vi "ELVIS III v1.0 Build MUX Configuration AI Continuous.vi"(11 "AI (Continuous) Channels List":T4) -> (2 "Bank Count":u8[](array[numeric]), 3 "Channel Reservation Info":T1)   [LabVIEW 2021]
uses:
  <vilib>/myRIO/Common/Instrument Driver Framework/ELVIS III v1.0/AI Continuous/typedefs/AI Continuous Channels List.ctl
  <vilib>/myRIO/Common/Instrument Driver Framework/ELVIS III v1.0/AI Continuous/typedefs/ELVIS III v1.0 AI Continuous Channels Enum.ctl
  <vilib>/myRIO/Common/Instrument Driver Framework/ELVIS III v1.0/Resource Manager/typedefs/ELVIS III v1.0 Channel Reservation List.ctl
  <vilib>/myRIO/Common/Instrument Driver Framework/ELVIS III v1.0/Resource Manager/typedefs/ELVIS III v1.0 Channel Reservation Info.ctl
  <vilib>/myRIO/Common/Instrument Driver Framework/ELVIS III v1.0/Resource Manager/typedefs/ELVIS III v1.0 Connector List.ctl
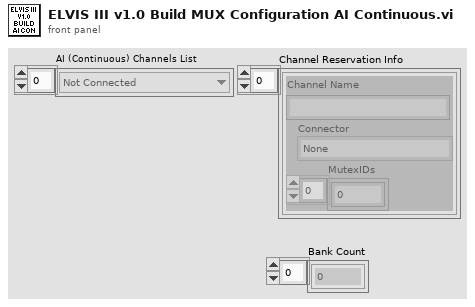
[diagram p1: front panel]
types:
  T1 = typedef "ELVIS III v1.0 Channel Reservation List.ctl" = T2[]
  T2 = typedef "ELVIS III v1.0 Channel Reservation Info.ctl" = cluster{"Channel Name":string, "Connector":T3, "MutexIDs":u32[]}
  T3 = typedef "ELVIS III v1.0 Connector List.ctl" = enum32{"None", "ConnectorA", "ConnectorB"}
  T4 = typedef "AI Continuous Channels List.ctl" = T5[]
  T5 = typedef "ELVIS III v1.0 AI Continuous Channels Enum.ctl" = enum16{"Not Connected", "A/AI0 (Continuous)", "A/AI1 (Continuous)", "A/AI2 (Continuous)", "A/AI3 (Continuous)", "A/AI4 (Continuous)", "A/AI5 (Continuous)", "A/AI6 (Continuous)", "A/AI7 (Continuous)", "A/AI0 (DIFF Continuous)", "A/AI1 (DIFF Continuous)", "A/AI2 (DIFF Continuous)", "A/AI3 (DIFF Continuous)", "B/AI0 (Continuous)", "B/AI1 (Continuous)", "B/AI2 (Continuous)", "B/AI3 (Continuous)", "B/AI4 (Continuous)", "B/AI5 (Continuous)", "B/AI6 (Continuous)", "B/AI7 (Continuous)", "B/AI0 (DIFF Continuous)", "B/AI1 (DIFF Continuous)", "B/AI2 (DIFF Continuous)", "B/AI3 (DIFF Continuous)"}
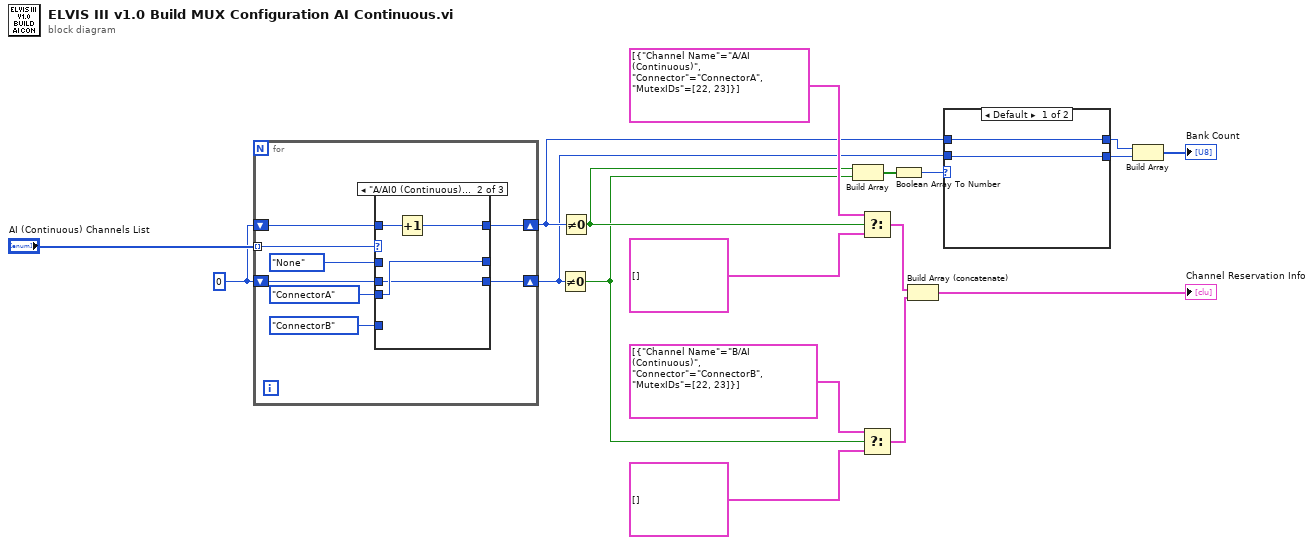
[diagram p0: block diagram]
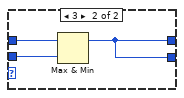
[diagram p2: hidden frame]
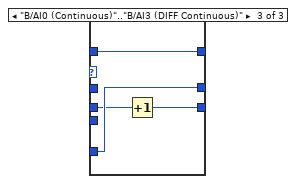
[diagram p4: hidden frame]
diagram:
  w10 = u8 0
  n1 = for {
    tunnel: "AI (Continuous) Channels List" -> [w26] mode=indexing
    shift-right: [w21] -> w5
    shift-left: w10 -> [w22]
    shift-right: [w19] -> w4
    shift-left: w10 -> [w20]
    n2 = case shown="\"A/AI0 (Continuous)\"..\"A/AI3 (DIFF Continuous)\"" w26 {
      tunnel: ELVIS_III_v1.0_Connector_List."None" ("Connector") -> [w29 _ _]
      tunnel: [w29 w33 w37] -> _
      tunnel: ELVIS_III_v1.0_Connector_List."ConnectorA" ("Connector") -> [_ w33 _]
      tunnel: ELVIS_III_v1.0_Connector_List."ConnectorB" ("Connector") -> [_ _ w37]
      tunnel: w22 -> [w28 w31 w36]
      tunnel: [w28 w30 w36] -> w21
      tunnel: w20 -> [w27 w32 w35]
      tunnel: [w27 w32 w34] -> w19
      frame "Not Connected", Default {
      }
      frame "A/AI0 (Continuous)".."A/AI3 (DIFF Continuous)" {
        n3 = Increment(x=w31) -> (x+1=w30:u8)
      }
      frame "B/AI0 (Continuous)".."B/AI3 (DIFF Continuous)" {
        n4 = Increment(x=w35) -> (x+1=w34:u8)
      }
    }
  }
  n5 = Not Equal To 0?(x=w4) -> (x != 0?=w7:bool)
  n6 = Not Equal To 0?(x=w5) -> (x != 0?=w8:bool)
  n7 = Build Array(w8, w7) -> (w9:bool[])
  n8 = Select(t=T2[] [{"Channel Name"="A/AI (Continuous)", "Connector"=enum."ConnectorA", "MutexIDs"=[22, 23]}], s=w8, f=T2[] []) -> (s? t:f=w15:T2[])
  n9 = Select(t=T2[] [{"Channel Name"="B/AI (Continuous)", "Connector"=enum."ConnectorB", "MutexIDs"=[22, 23]}], s=w7, f=T2[] []) -> (s? t:f=w12:T2[])
  n10 = Boolean Array To Number(Boolean array=w9) -> (number=w6:u32)
  n11 = Build Array (concatenate)(w15, w12) -> (→"Channel Reservation Info":T2[])
  n12 = case shown="Default" w6 {
    tunnel: w5 -> [w39 w42]
    tunnel: w4 -> [w38 w41]
    tunnel: [w39 w40] -> w3
    tunnel: [w38 w40] -> w2
    frame Default {
    }
    frame 3 {
      n13 = Max & Min(x=w42, y=w41) -> (max(x,y)=w40:u8)  [unwired: 1 out]
    }
  }
  n14 = Build Array(w3, w2) -> (→"Bank Count":u8[])
